vi "BCtr6b.vi"() -> ()   [LabVIEW 2016]
uses:
  <vilib>/Platform/TimedLoop/XDataNode/timing_clust.ctl
  <vilib>/Platform/TimedLoop/XDataNode/nitl_modes.ctl
  <vilib>/Platform/TimedLoop/XDataNode/wakeup.ctl
  <vilib>/platform/TimedLoop/XDataNode/XDataNode.xnode
  <vilib>/Platform/TimedLoop/XDataNode/XDNodeRunTimeDep.lvlib
panel:
  out "XY Graph":cluster{"Time":dbl[], dbl[]}(graph)
  in  "stop":bool
  out "LoopCt":dbl
  out "Ack":bool
  out "error out":errorcluster
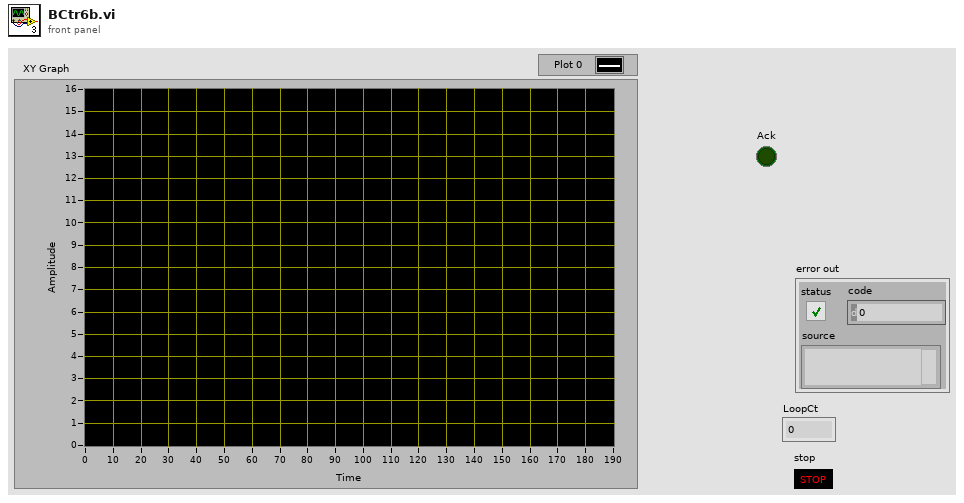
[diagram p1: front panel]
types:
  T1 = cluster{"Nbins":u16, "BaseAddrOut":u16, "PortOut":string, "ConfigOK":bool, "MreadFmt":string, "Time":dbl[], "Weight":dbl[]}
  T2 = typedef "XDNodeRunTimeDep.lvlib/timing_clust.ctl" = cluster{"Expected End [f-1]":u64, "Actual End [f-1]":u64, "Finished Late? [f-1]":bool, "Expected End [i-1]":u64, "Actual End [i-1]":u64, "Finished Late? [i-1]":bool, "Expected Start [i]":u64, "Actual Start [i]":u64, "Expected Start [f]":u64, "Actual Start [f]":u64, "Source Name":string, "Structure Name":string, "Period":i64, "Deadline":i64, "Offset":i64, "Start":i64, "Priority":i32, "Timeout":i32, "Mode":T3, "Wakeup Reason":T4, "Error":errorcluster, "Source Type":string, "Secondary Source Type":string, "Global End Time":u64, "Global Start Time":u64, "Frame Duration":u64, "Iteration Duration":u64, "Assigned CPU":i32, "I/O Scan Engine Mode":u32}
  T3 = typedef "XDNodeRunTimeDep.lvlib/nitl_modes.ctl" = enum32{"No Change", "Process missed periods, maintain original phase", "Discard missed periods, maintain original phase", "Process missed periods, ignore original phase", "Discard missed periods, ignore original phase"}
  T4 = typedef "XDNodeRunTimeDep.lvlib/wakeup.ctl" = enum32{"Normal", "Aborted", "Asynchronous wakeup", "Timing source error", "Timed loop error", "Timeout"}
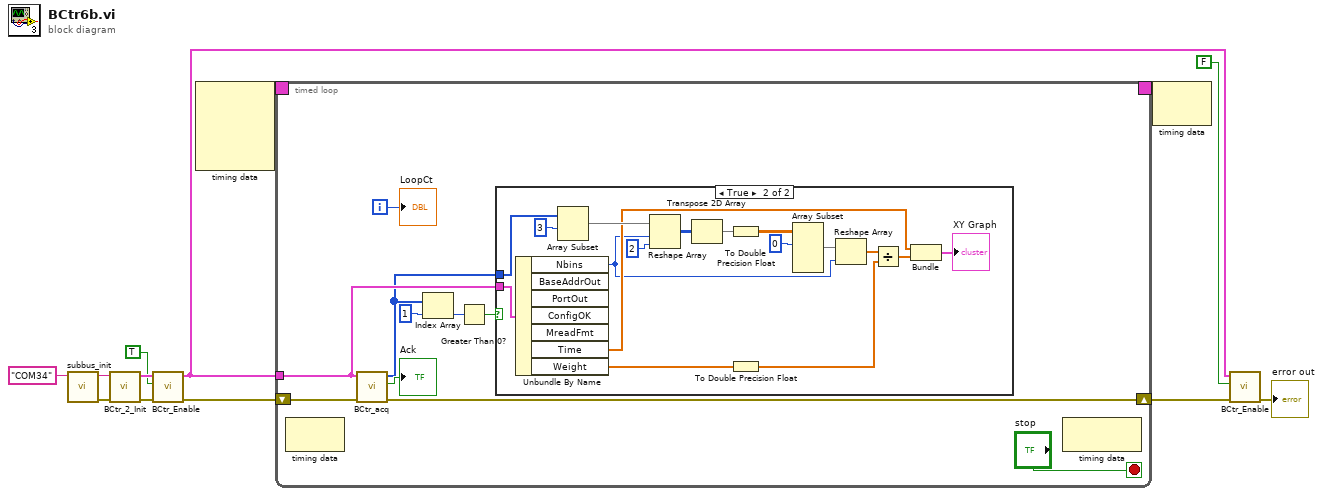
[diagram p0: block diagram]
diagram:
  n1 = call "subbus_init.vi"("Port"="COM34") -> ("error out"=w9:errorcluster, "PortOut"=w10:string)  [unwired: 9 in]
  n2 = call "BCtr_2_Init.vi"("error in (no error)"=w9, "SBPort"=w10) -> ("error out"=w7:errorcluster, "CtrCfg"=w8:T1)  [unwired: 8 in]
  n3 = call "BCtr_Enable.vi"("error in (no error)"=w7, "Enable"=TRUE, "CtrCfg"=w8) -> ("error out"=w6:errorcluster, "CtrCfg"=w2:T1)  [unwired: 5 in, 1 out]
  n4 = node-c288() -> (w12:T2)  [unwired: 4 in]
  n5 = timed-loop {
    timing: w12 -> [_]
    timing-out: [_] -> w11
    shift-right: [w22] -> w4
    shift-left: w6 -> [w23]
    tunnel: w2 -> [w18]
    i -> [w20]
    stop <- "stop" stop-if-true
    n6 = node-c288() -> ()  [unwired: 1 in, 1 out]
    n7 = call "BCtr_acq.vi"("error in (no error)"=w23, "CtrCfg"=w18) -> ("error out"=w22:errorcluster, "Ack"=→"Ack":bool, "Values"=w16:u16[])  [unwired: 7 in]
    n8 = Index Array(array=w16, index=1) -> (element=w17:u16)
    n9 = Greater Than 0?(x=w17) -> (x > 0?=w14:bool)
    n10 = case shown="True" w14 {
      tunnel: w18 -> [_ w38]
      tunnel: w16 -> [_ w24]
      frame False {
      }
      frame True {
        n11 = Unbundle By Name(w38) -> ("Nbins"=w25:u16, "Time"=w35:dbl[], "Weight"=w32:dbl[])  [unwired: 4 out]
        n12 = Array Subset(array=w24, index=3) -> (w39:u16[])  [unwired: 1 in]
        n13 = Reshape Array(w39, w25, 2) -> (w36:u16[][])
        n14 = Transpose 2D Array(2D array=w36) -> (transposed array=w33:u16[][])
        n15 = To Double Precision Float(number=w33) -> (double precision float=w30:dbl[][])
        n16 = To Double Precision Float(number=w32) -> (double precision float=w31:dbl[])
        n17 = Array Subset(array=w30, index (row)=0) -> (w28:dbl[][])  [unwired: 3 in]
        n18 = Reshape Array(w28, w25) -> (w27:dbl[])
        n19 = Divide(x=w27, y=w31) -> (x/y=w34:dbl[])
        n20 = Bundle("Time"=w35, w34) -> (→"XY Graph":cluster{"Time":dbl[], dbl[]})  [unwired: 1 in]
      }
    }
    n21 = node-c288() -> ()  [unwired: 1 in, 1 out]
    "LoopCt" <- w20
  }
  n22 = node-c288(w11) -> ()  [unwired: 1 out]
  n23 = call "BCtr_Enable.vi"("error in (no error)"=w4, "Enable"=FALSE, "CtrCfg"=w2) -> ("error out"=→"error out":errorcluster)  [unwired: 5 in, 2 out]
